vi "FX2 VISA Com.vi"(4 "error in (no error)":errorcluster, 5 "VISA Resource":refnum<visa-resource-name>) -> (1 "error out":errorcluster)   [LabVIEW 2015]
uses:
  MARS_Global_var.vi
panel:
  out "Delimeter":string
  out "ByteCount":string
  out "Address":string
  out "RecordType":string
  out "Data":string
  out "NumberOfBytes":u32
  in  "Load Hex file":path
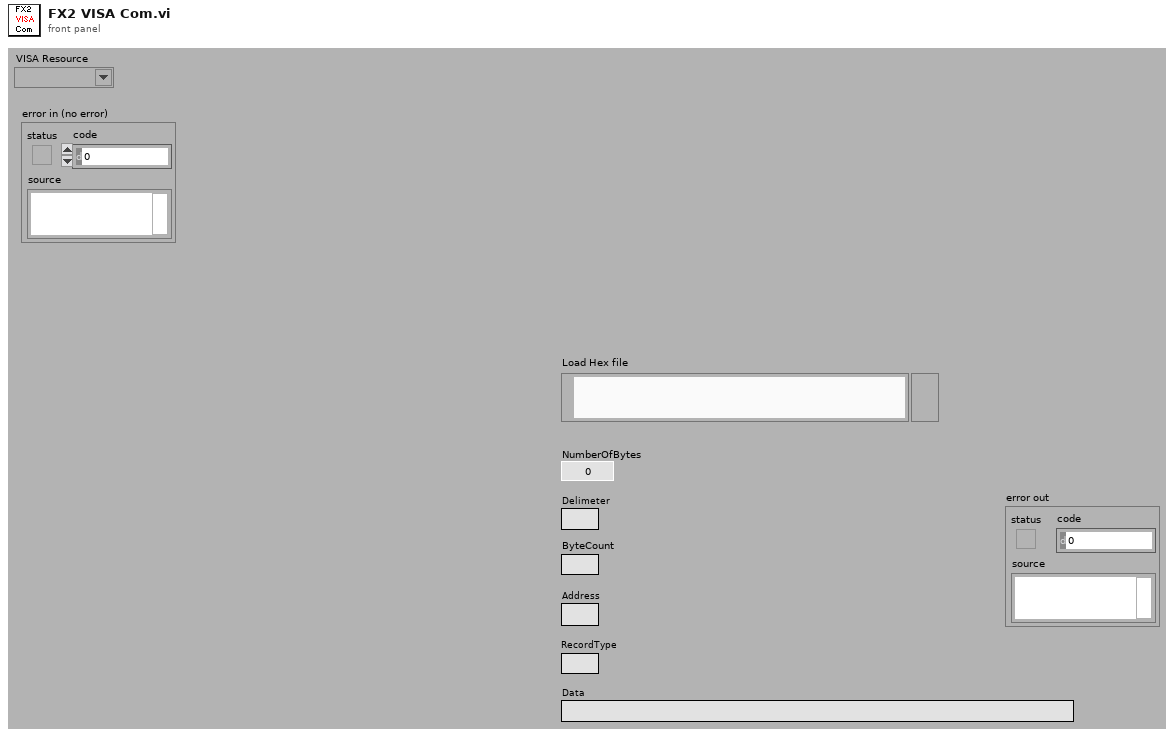
[diagram p1: front panel]
types:
  T1 = enum16{"open", "replace", "create", "open or create", "replace or create", "replace or create with confirmation"}
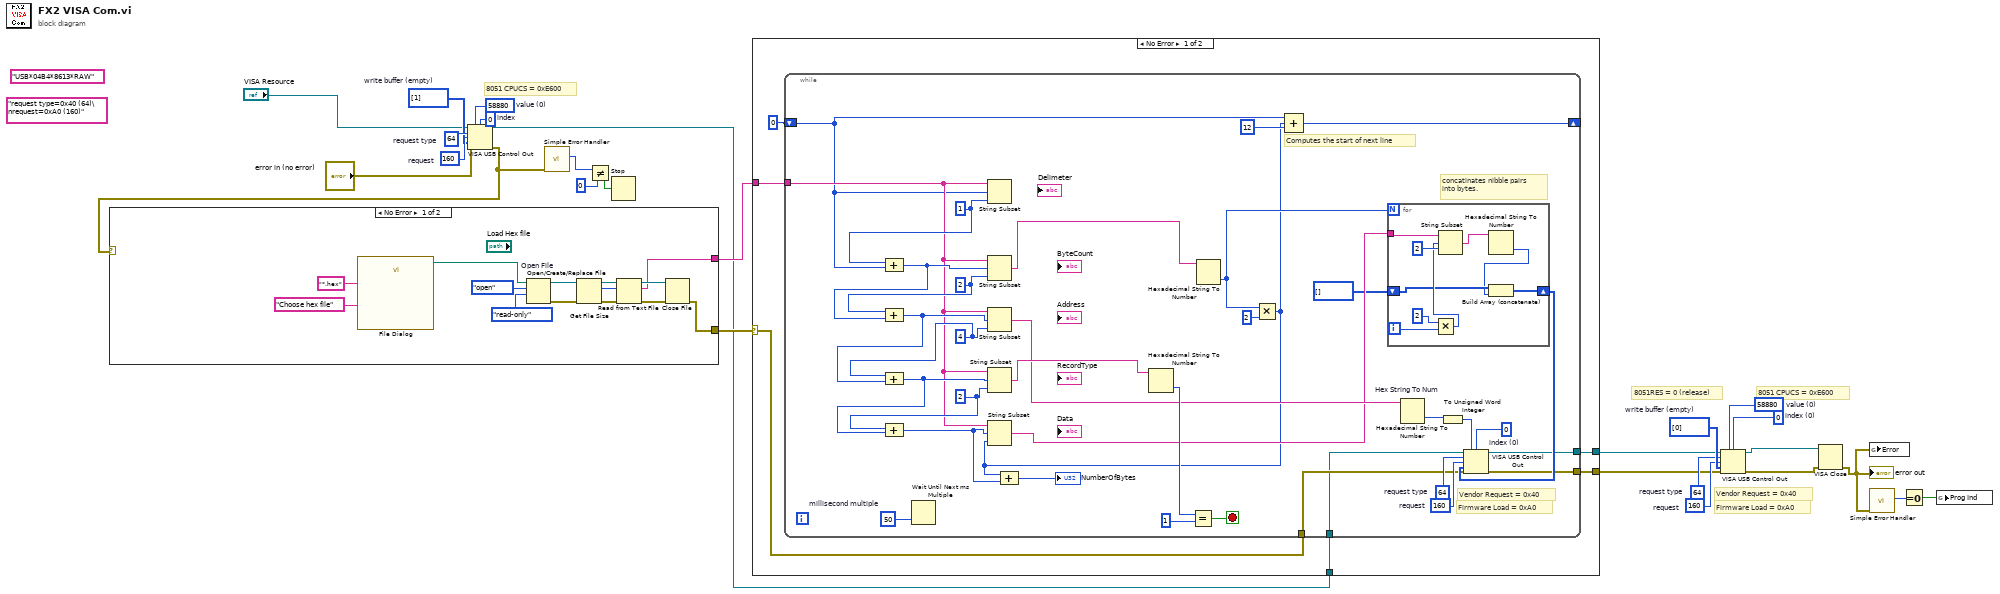
[diagram p0: block diagram]
diagram:
  (unwired) "USB*04B4*8613*RAW"
  (unwired) "request type=0x40 (64)\nrequest=0xA0 (160)"
  w12 = u8[] [1]  # write buffer (empty)
  w19 = u16 0  # index (0)
  w18 = u16 58880  # value (0)
  w17 = u8[] [0]  # write buffer (empty)
  w16 = i16 160  # request
  w15 = i16 64  # request type
  w23 = u16 58880  # value (0)
  w24 = 64  # request type
  w26 = 0  # index
  w25 = 160  # request
  # "8051RES = 0 (release)"
  # "Firmware Load = 0xA0"
  # "Vendor Request = 0x40"
  # "8051 CPUCS = 0xE600"
  # "8051 CPUCS = 0xE600"
  n1 = VISA USB Control Out(0:"VISA Resource", 1:w23, 2:w26, 5:w24, 7:w25, 9:w12, 11:"error in (no error)") -> (4:w20:refnum<visa-resource-name>, 15:w9:errorcluster)
  n2 = case shown="No Error" w9 {
    selector: w9 -> [_ w41]
    tunnel: [w31 w41] -> w22
    tunnel: [w30 _] -> w21
    frame No Error {
      n3 = call "File Dialog"("prompt"="Choose hex file", "pattern (all files)"="*.hex") -> ("selected path"=w27:path)  [unwired: 10 in, 3 out]
      n4 = Open/Create/Replace File "Open File"(file path (use dialog)=w27, operation (0:open)=T1."open", access (0:read/write)=enum16{"read/write", "read-only", "write-only"}."read-only") -> (refnum out=w34:refnum<file>, error out=w35:errorcluster)  [unwired: 3 in, 1 out]
      n5 = Get File Size(file=w34, error in=w35) -> (refnum out=w36:refnum<file>, size (in bytes)=w40:i64, 0:w37:errorcluster)
      n6 = Read from Text File(file (use dialog)=w36, count=w40, error in=w37) -> (refnum out=w38:refnum<file>, text=w30:string, error out=w39:errorcluster)  [unwired: 1 in, 1 out]
      n7 = Close File(refnum=w38, error in=w39) -> (error out=w31:errorcluster)  [unwired: 1 out]
    }
    frame Error {
    }
  }
  n8 = call <vilib>:"Simple Error Handler.vi"("error in (no error)"=w9) -> ("code out"=w8:i32)  [unwired: 4 in, 4 out]
  n9 = Not Equal?(x=w8, y=0) -> (x != y?=w10:bool)
  n10 = Stop(stop? (T)=w10) -> ()
  n11 = case shown="No Error" w22 {
    selector: w22 -> [w44 w93]
    tunnel: [w45 w93] -> w13
    tunnel: [w46 w92] -> w14
    tunnel: w21 -> [w43 _]
    tunnel: w20 -> [w42 w92]
    frame No Error {
      n12 = while {
        shift-right: [w77] -> _
        shift-left: u32 0 -> [w48]
        tunnel: w43 -> [w53]
        tunnel: [w52] -> w46
        tunnel: [w51] -> w45
        tunnel: w44 -> [w50]
        tunnel: w42 -> [w49]
        stop <- w81 stop-if-true
        w64 = u16 0  # index (0)
        w65 = i16 160  # request
        w66 = i16 64  # request type
        w67 = u32 50  # millisecond multiple
        w69 = 2 ("length (rest)")
        w71 = 4 ("length (rest)")
        w73 = 2 ("length (rest)")
        w75 = 1 ("length (rest)")
        # "Computes the start of next line"
        # "Firmware Load = 0xA0"
        # "Vendor Request = 0x40"
        # "concatinates nibble pairs\ninto bytes."
        n13 = Compound Arithmetic op=ADD(w75, w48) -> (w74:u32)
        n14 = Compound Arithmetic op=ADD(w74, w73) -> (w72:u32)
        n15 = Compound Arithmetic op=ADD(w72, w71) -> (w70:u32)
        n16 = Compound Arithmetic op=ADD(w70, w69) -> (w55:u32)
        n17 = Wait Until Next ms Multiple(millisecond multiple=w67) -> ()  [unwired: 1 out]
        n18 = String Subset(string=w53, offset (0)=w48, length (rest)=w75) -> ()  [unwired: 1 out]
        n19 = String Subset(string=w53, offset (0)=w74, length (rest)=w73) -> (substring=w78:string)
        n20 = String Subset(string=w53, offset (0)=w72, length (rest)=w71) -> (substring=w63:string)
        n21 = String Subset(string=w53, offset (0)=w70, length (rest)=w69) -> (substring=w80:string)
        n22 = Hexadecimal String To Number(string=w80) -> (number=w79:u32)  [unwired: 2 in, 1 out]
        n23 = Equal?(x=w79, y=u32 1) -> (x = y?=w81:bool)
        n24 = Hexadecimal String To Number(string=w78) -> (number=w59:u32)  [unwired: 2 in, 1 out]
        n25 = Multiply(x=w59, y=u32 2) -> (x*y=w54:u32)
        n26 = String Subset(string=w53, offset (0)=w55, length (rest)=w54) -> (substring=w60:string)
        n27 = Compound Arithmetic op=ADD(w54, w55) -> (→"NumberOfBytes":u32)
        n28 = Compound Arithmetic op=ADD(w48, w54, u32 12 ("value")) -> (w77:u32)
        n29 = for {
          N: w59 -> [_]
          tunnel: w60 -> [w91]
          shift-right: [w84] -> w57
          shift-left: u32[] [] -> [w85]
          i -> [w88]
          n30 = Multiply(x=2, y=w88) -> (x*y=w87:i32)
          n31 = String Subset(string=w91, offset (0)=w87, length (rest)=2 ("length (rest)")) -> (substring=w89:string)
          n32 = Hexadecimal String To Number(string=w89) -> (number=w83:u32)  [unwired: 2 in, 1 out]
          n33 = Build Array (concatenate) "Build Array"(w85, w83) -> (w84:u32[])
        }
        n34 = Hexadecimal String To Number "Hex String To Num"(string=w63) -> (number=w62:u32)  [unwired: 2 in, 1 out]
        n35 = To Unsigned Word Integer(number=w62) -> (unsigned 16bit integer=w61:u16)
        n36 = VISA USB Control Out(0:w49, 1:w61, 2:w64, 5:w66, 7:w65, 9:w57, 11:w50) -> (4:w52:refnum<visa-resource-name>, 15:w51:errorcluster)
      }
    }
    frame Error {
    }
  }
  n37 = VISA USB Control Out(0:w14, 1:w18, 2:w19, 5:w15, 7:w16, 9:w17, 11:w13) -> (4:w6:refnum<visa-resource-name>, 15:w5:errorcluster)
  n38 = VISA Close(VISA resource name=w6, error in (no error)=w5) -> (error out=w3:errorcluster)
  "error out" <- w3
  n39 = global write "MARS_Global_var.vi" "Error"(w3) -> ()
  n40 = call <vilib>:"Simple Error Handler.vi"("error in (no error)"=w3) -> ("code out"=w7:i32)  [unwired: 4 in, 4 out]
  n41 = Equal To 0?(x=w7) -> (x = 0?=w4:bool)
  n42 = global write "MARS_Global_var.vi" "Prog Ind"(w4) -> ()
